vi "SnapToPoint.vi"(9 "Cursor.Cursor Position in":T1, 11 "Value":cluster{"x0":dbl, "df":dbl, dbl[]}[](array[cluster])) -> (1 "Cursor.Cursor Position out":T1)   [LabVIEW 2022 SP3]
uses:
  <vilib>/Utility/miscctls.llb/LVPointDoubleTypeDef.ctl
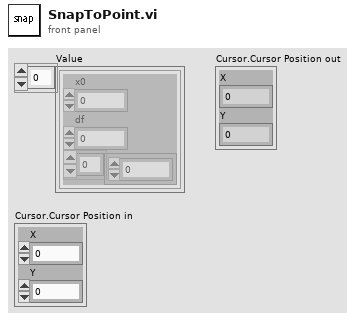
[diagram p1: front panel]
types:
  T1 = typedef "LVPointDoubleTypeDef.ctl" = cluster{"X":dbl, "Y":dbl}
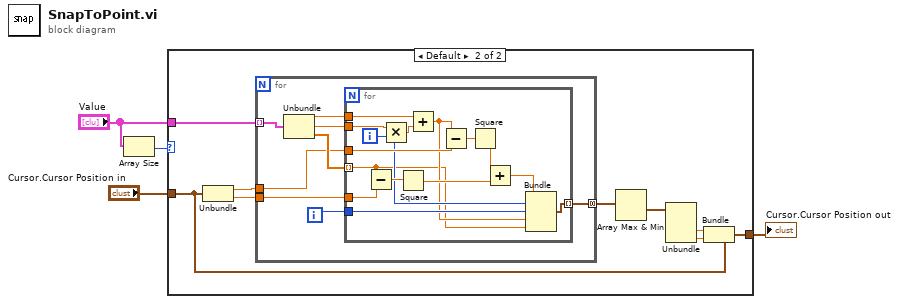
[diagram p0: block diagram]
diagram:
  n1 = Array Size(array="Value") -> (size(s)=w1:i32)
  n2 = case shown="Default" w1 {
    tunnel: "Cursor.Cursor Position in" -> [w5 w6]
    tunnel: [w5 w8] -> w3
    tunnel: "Value" -> [_ w7]
    frame 0 {
    }
    frame Default {
      n3 = Unbundle(w6) -> ("X"=w13:dbl, "Y"=w14:dbl)
      n4 = for {
        tunnel: w7 -> [w22] mode=indexing
        tunnel: w14 -> [w18]
        tunnel: w13 -> [w17]
        tunnel: [w15] -> w12 mode=concatenating
        i -> [w16]
        n5 = Unbundle(w22) -> ("x0"=w19:dbl, "df"=w20:dbl, w21:dbl[])
        n6 = for {
          tunnel: w21 -> [w23] mode=indexing
          tunnel: w20 -> [w37]
          tunnel: w19 -> [w35]
          tunnel: w18 -> [w34]
          tunnel: w17 -> [w32]
          tunnel: w16 -> [w26]
          tunnel: [w25] -> w15 mode=indexing
          i -> [w27]
          n7 = Subtract(x=w23, y=w34) -> (x-y=w33:dbl)
          n8 = Multiply(x=w37, y=w27) -> (x*y=w36:dbl)
          n9 = Square(x=w33) -> (x^2=w29:dbl)
          n10 = Add(x=w35, y=w36) -> (x+y=w24:dbl)
          n11 = Subtract(x=w24, y=w32) -> (x-y=w31:dbl)
          n12 = Square(x=w31) -> (x^2=w30:dbl)
          n13 = Add(x=w30, y=w29) -> (x+y=w28:dbl)
          n14 = Bundle(w28, w27, w26, w24, w23) -> (w25:cluster{dbl, i32, i32, dbl, dbl})  [unwired: 1 in]
        }
      }
      n15 = Array Max & Min(array=w12) -> (min value=w11:cluster{dbl, i32, i32, dbl, dbl})  [unwired: 3 out]
      n16 = Unbundle(w11) -> (w10:dbl, w9:dbl)  [unwired: 3 out]
      n17 = Bundle(cluster=w6, "X"=w10, "Y"=w9) -> (w8:T1)
    }
  }
  "Cursor.Cursor Position out" <- w3
